vi "Insert into IOCONFIG.vi"(8 "error in (no error)":errorcluster, 9 "IO Type":string="AI", 10 "AI in":string[][](array[string]), 11 "connection reference":T1) -> (0 "error out":errorcluster)   [LabVIEW 2018]
uses:
  <vilib>/addons/database/Connection.llb/Conn ObjectReference.ctl
  <vilib>/addons/database/Connection.llb/Conn Execute.vi
  <vilib>/addons/database/Recordset.llb/Rec Destroy - Connection.vi
  <vilib>/addons/database/NI_Database_API.lvlib
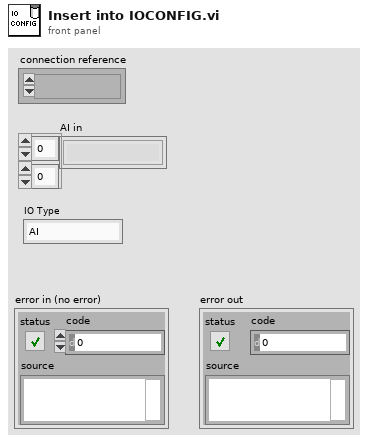
[diagram p1: front panel]
types:
  T1 = typedef "NI_Database_API.lvlib/Conn ObjectReference.ctl" = refnum<k1>
  T2 = typedef "NI_Database_API.lvlib/Rec ObjectReference.ctl" = refnum<k1>
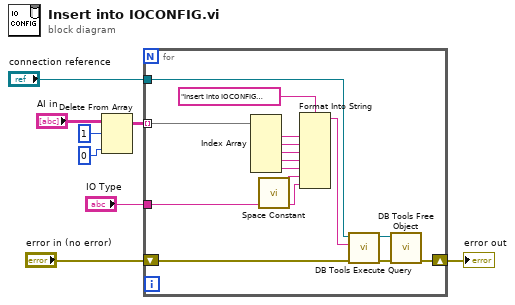
[diagram p0: block diagram]
diagram:
  n1 = Delete From Array(array="AI in", length=1, index (col)=0 ("disabled index (col)")) -> (array with subset deleted=w2:string[][])  [unwired: 1 in, 1 out]
  n2 = for {
    tunnel: w2 -> [w22] mode=indexing
    tunnel: "connection reference" -> [w23]
    shift-right: [w10] -> w7
    shift-left: "error in (no error)" -> [w11]
    tunnel: "IO Type" -> [w9]
    n3 = Index Array(array=w22) -> (element #1=w20:string, element #2=w19:string, element #3=w18:string, element #4=w17:string, element #5=w16:string)  [unwired: 5 in]
    n4 = call <vilib>:"Space Constant.vi"() -> ("String"=w15:string)
    n5 = Format Into String(format string="Insert into IOCONFIG  VALUES('%s','%s','%s','%s','%s','%s','%s')", w20, w19, w18, w17, w16, w15, w9) -> (resulting string=w14:string)  [unwired: 2 in, 1 out]
    n6 = call-poly <vilib>:"DB Tools Execute Query.vi"("error in (no error)"=w11, "SQL query"=w14, "connection reference"=w23) -> ("error out"=w13:errorcluster, "recordset reference"=w12:T2)  [unwired: 5 in]
    n7 = call-poly <vilib>:"DB Tools Free Object.vi"("error in (no error)"=w13, "recordset reference"=w12) -> ("error out"=w10:errorcluster)  [unwired: 8 in, 1 out]
  }
  "error out" <- w7
